vi "Echo Detector.vi"() -> ()   [LabVIEW 2020]
doc: "This example demonstrates how to detect echoes in a signal using the Fast Hilbert Transform VI."
uses:
  <vilib>/Analysis/NI_AALPro.lvlib
panel:
  in  "Amplitude":dbl(slide)=0.2226890756302521 scale=0.0..0.5
  in  "Echo Amplitude":dbl(slide)=0.01680672268907563 scale=0.0..0.5
  in  "Decay Value":dbl(slide)=54.54545454545455 scale=0.0..100.0
  in  "Frequency":dbl(slide)=3.7373737373737375 scale=0.0..10.0
  out "Echoed Signal":dbl[](graph)
  out "Original Signal":dbl[](graph)
  in  "Echo Delay":i32(slide)=185 scale=50.0..200.0
  out "Resulting Signal":dbl[](graph)
  out "Echogram":dbl[](graph)
  in  "Stop":bool
  # "Overview: This example demonstrates how to detect echoes in a signal using the Fast Hilbert Transform VI.\nRequirements: LabVIEW Full Development System\nInstructions:\n1. Run the VI and change the Amplitude, Echo Amplitude, Decay Value and Echo Delay. \n2. Verify that the Echogram will give you the time delay of the echo.\n3. Click Stop to stop the VI."
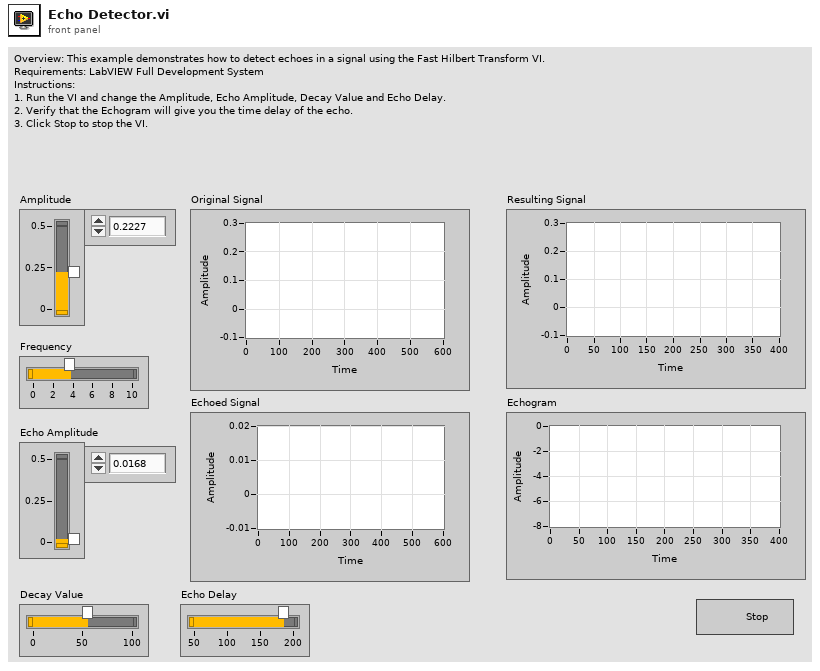
[diagram p1: front panel]
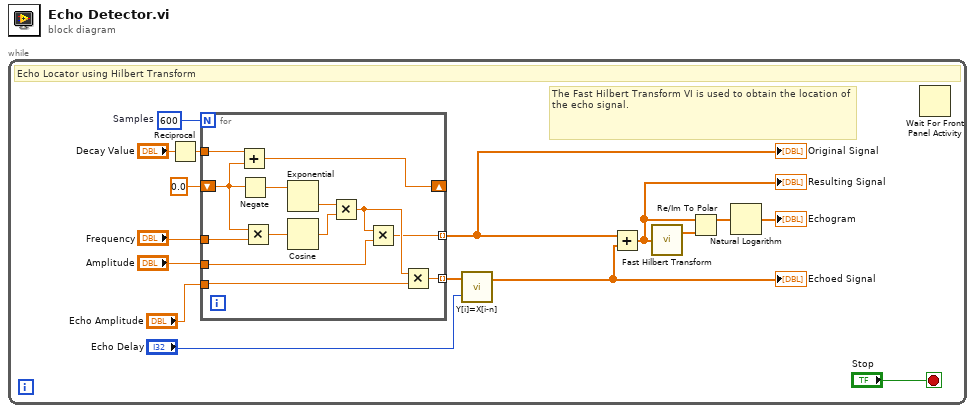
[diagram p0: block diagram]
diagram:
  n1 = while {
    stop <- "Stop" stop-if-true
    w9 = 600  # Samples
    # "The Fast Hilbert Transform VI is used to obtain the location of the echo signal."
    # "Echo Locator using Hilbert Transform"
    n2 = Reciprocal(x="Decay Value") -> (1/x=w13:dbl)
    n3 = for {
      N: w9 -> [_]
      shift-right: [w28] -> _
      shift-left: 0.0 -> [w26]
      tunnel: [w18] -> w7 mode=indexing
      tunnel: [w19] -> w14 mode=indexing
      tunnel: "Echo Amplitude" -> [w20]
      tunnel: "Amplitude" -> [w22]
      tunnel: "Frequency" -> [w27]
      tunnel: w13 -> [w29]
      n4 = Add(x=w29, y=w26) -> (x+y=w28:dbl)
      n5 = Negate(x=w26) -> (-x=w17:dbl)
      n6 = Multiply(x=w26, y=w27) -> (x*y=w25:dbl)
      n7 = Exponential(1:w17) -> (0:w23:dbl)
      n8 = Cosine(x=w25) -> (cos(x)=w24:dbl)
      n9 = Multiply(x=w23, y=w24) -> (x*y=w21:dbl)
      n10 = Multiply(x=w21, y=w22) -> (x*y=w18:dbl)
      n11 = Multiply(x=w21, y=w20) -> (x*y=w19:dbl)
    }
    "Original Signal" <- w7
    n12 = call <vilib>:"Y[i]=X[i-n].vi"("shifts: n"="Echo Delay", "Input Array"=w14) -> ("Shifted Array"=w6:dbl[])  [unwired: 1 out]
    "Echoed Signal" <- w6
    n13 = Add(x=w7, y=w6) -> (x+y=w10:dbl[])
    "Resulting Signal" <- w10
    n14 = call <vilib>:"Fast Hilbert Transform.vi"("X"=w10) -> ("Hilbert{X}"=w15:dbl[])  [unwired: 1 out]
    n15 = Re/Im To Polar(2:w15, 3:w10) -> (1:w16:dbl[])  [unwired: 1 out]
    n16 = Natural Logarithm(1:w16) -> (0:→"Echogram":dbl[])
    n17 = Wait For Front Panel Activity() -> ()  [unwired: 3 in, 1 out]
  }
